vi "Genius_game_mvp1.vi"() -> ()   [LabVIEW 2020]
doc: "Use this template to build a simple state machine design pattern. Each state executes code and determines which state to transition to."
uses:
  controls/Data.ctl
  Control 1.ctl
  <vilib>/numeric/Random Number (Range) I64.vi
  <vilib>/numeric/sub_Random U32.vi
panel:
  in  "Cancel Button":bool
  out "?":i32
  in  "Play":bool
  in  "?":T1
  out "?":u32(colorbox)
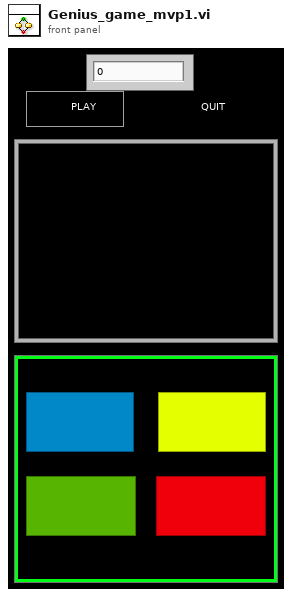
[diagram p1: front panel]
types:
  T1 = cluster{"BLUE":bool, "YELLOW":bool, "GREEN":bool, "RED":bool}
  T2 = typedef "Control 1.ctl" = enum32{"Play", "Initialise", "Create Colours", "Show colours sequence", "Wait for event", "pause", "Press colours sequence", "Compare colours", "Success ", "Failure", "Exit"}
  T3 = typedef "Data.ctl" = cluster{"Colours":i64[], "history ":i64[], "Wait time(ms)":u64, "String":string, "picked color":i64, "User's turn":i64, "Score":i64}
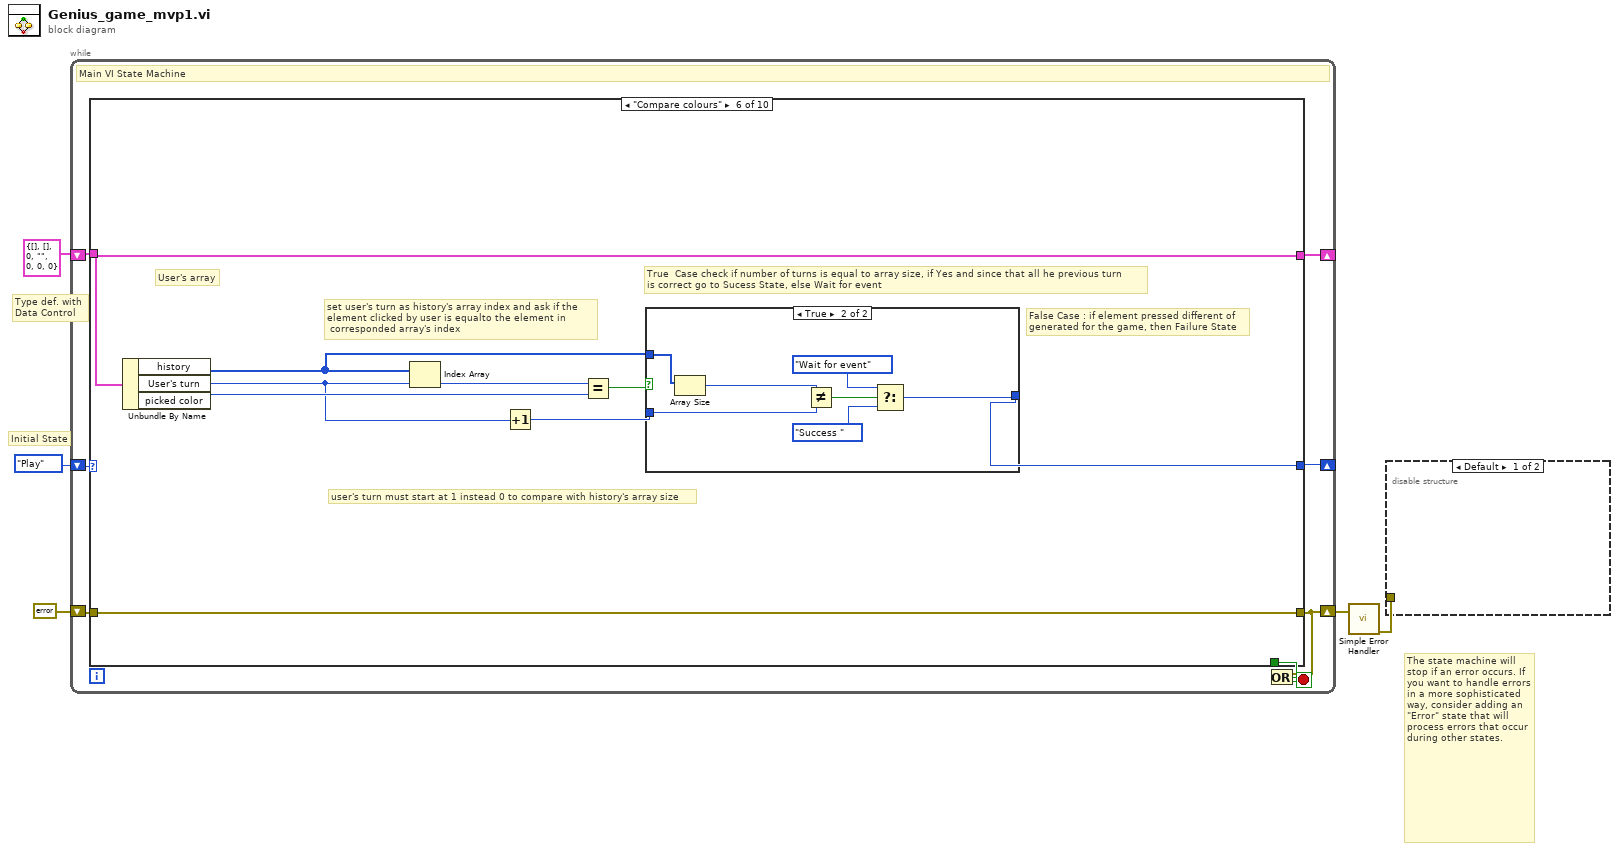
[diagram p0: block diagram]
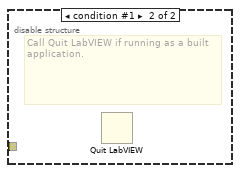
[diagram p2: hidden frame]
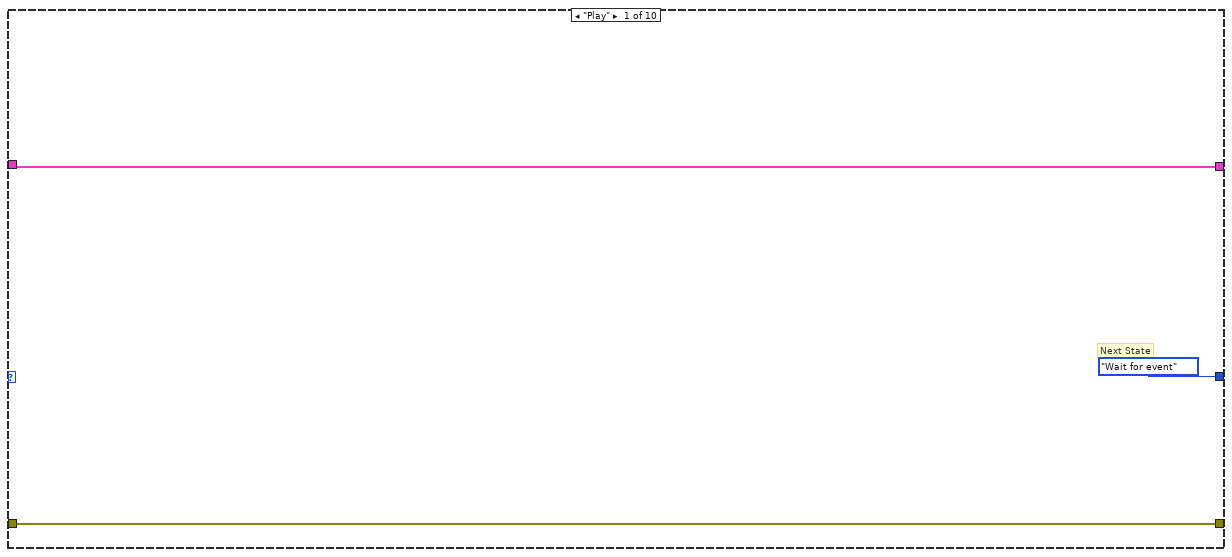
[diagram p3: hidden frame]
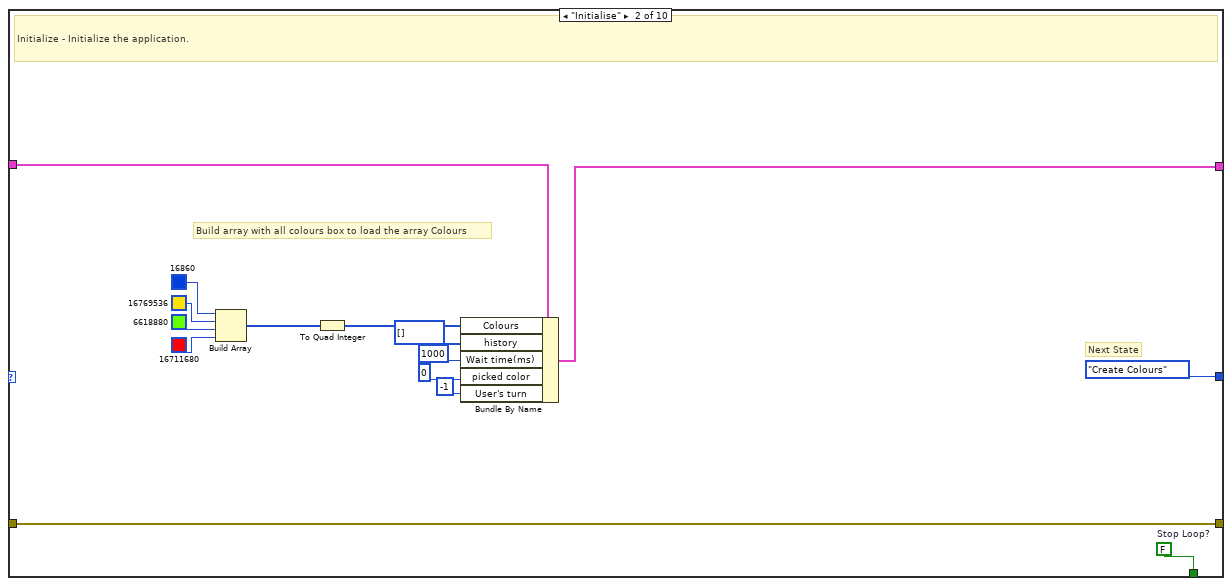
[diagram p4: hidden frame]
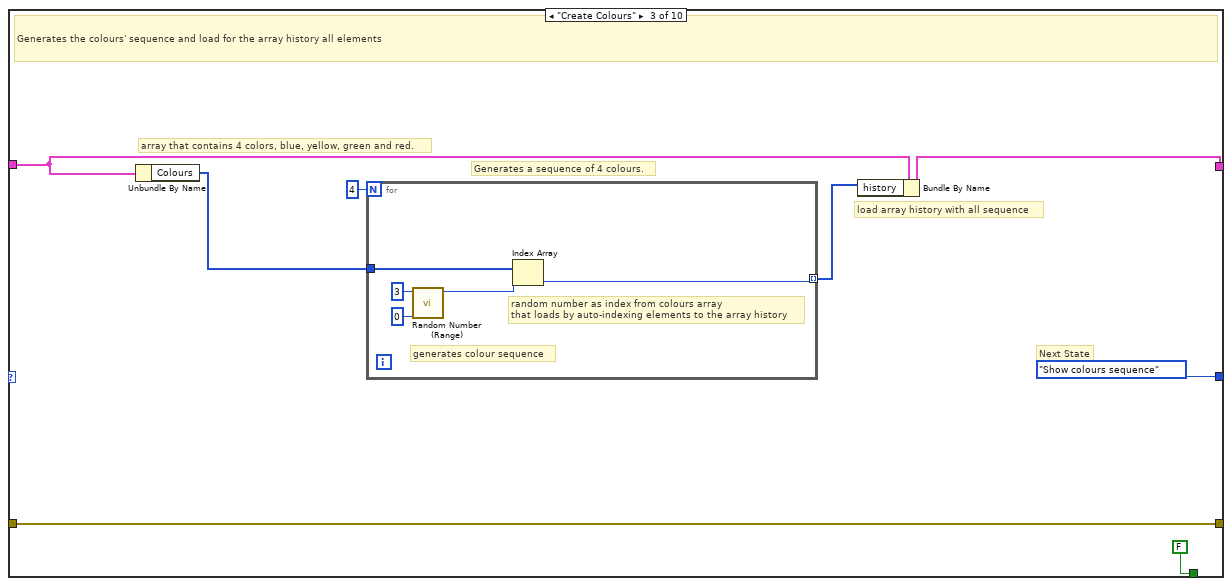
[diagram p5: hidden frame]
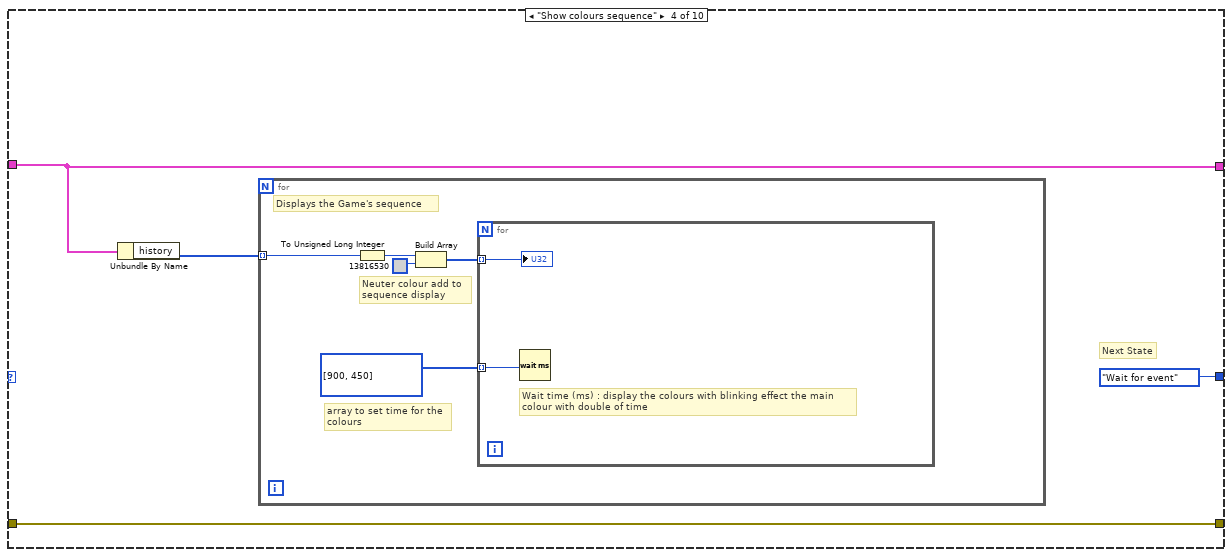
[diagram p6: hidden frame]
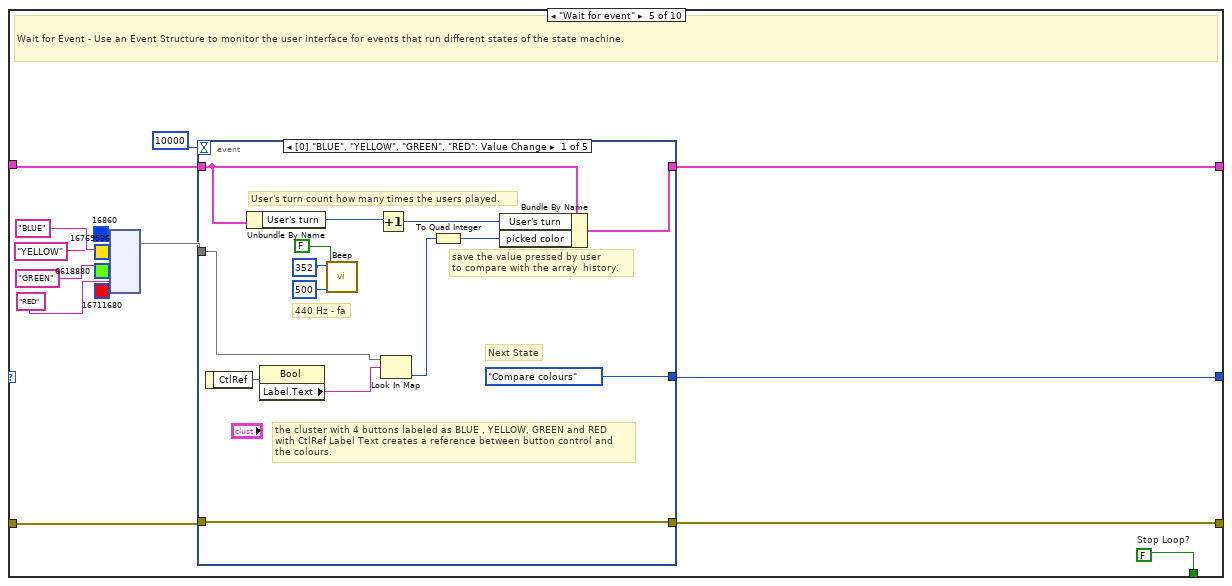
[diagram p7: hidden frame]
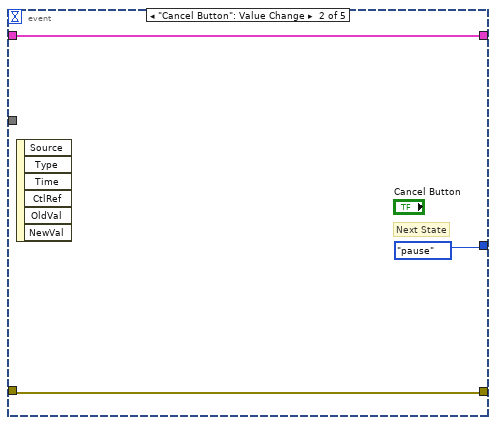
[diagram p8: hidden frame]
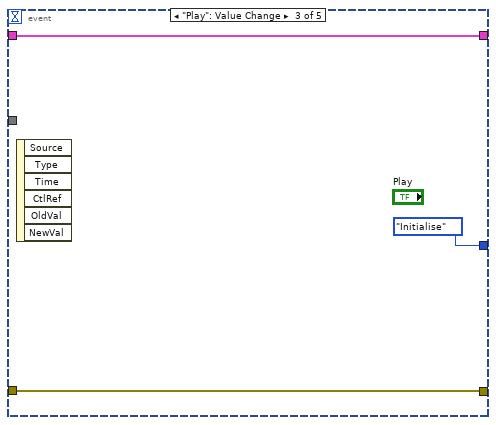
[diagram p9: hidden frame]
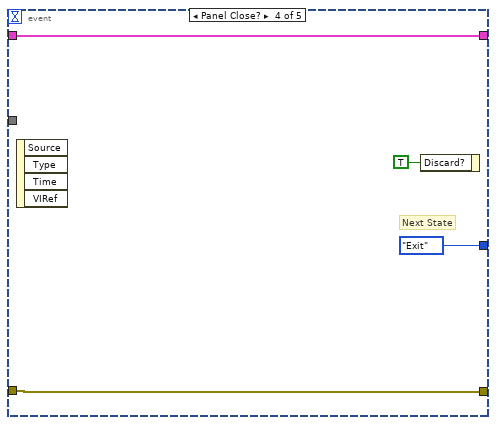
[diagram p10: hidden frame]
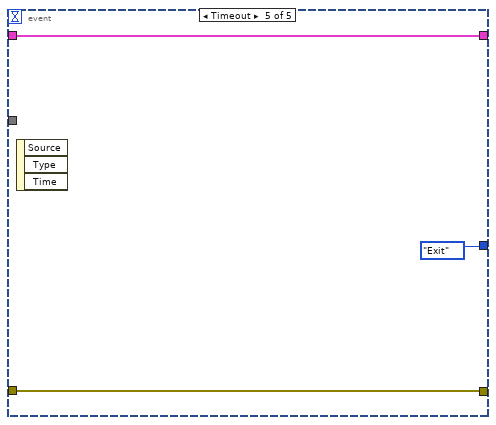
[diagram p11: hidden frame]
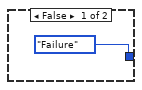
[diagram p12: hidden frame]
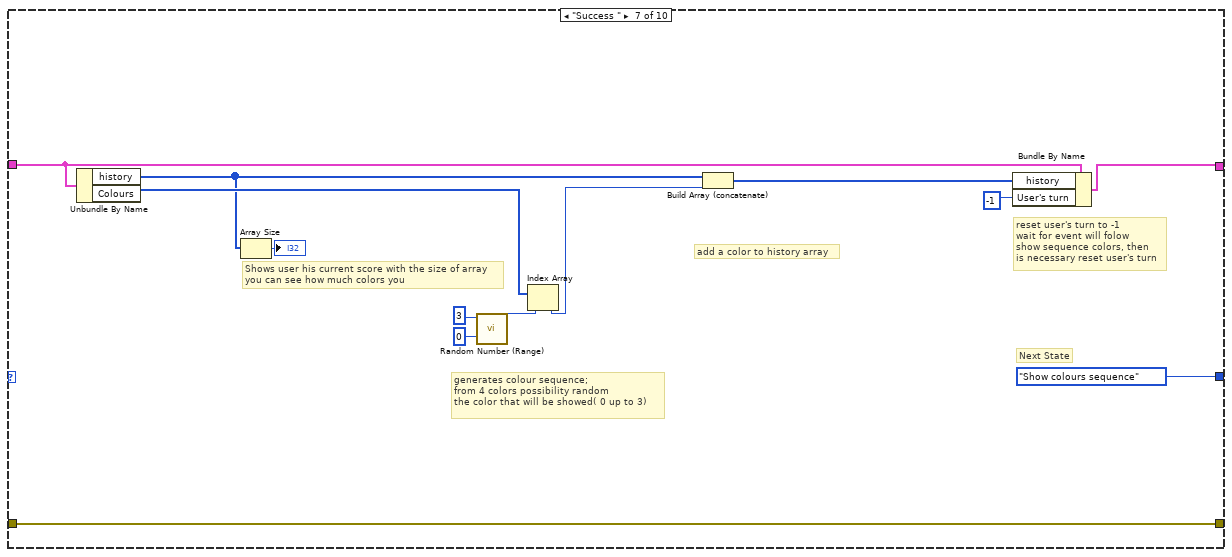
[diagram p13: hidden frame]
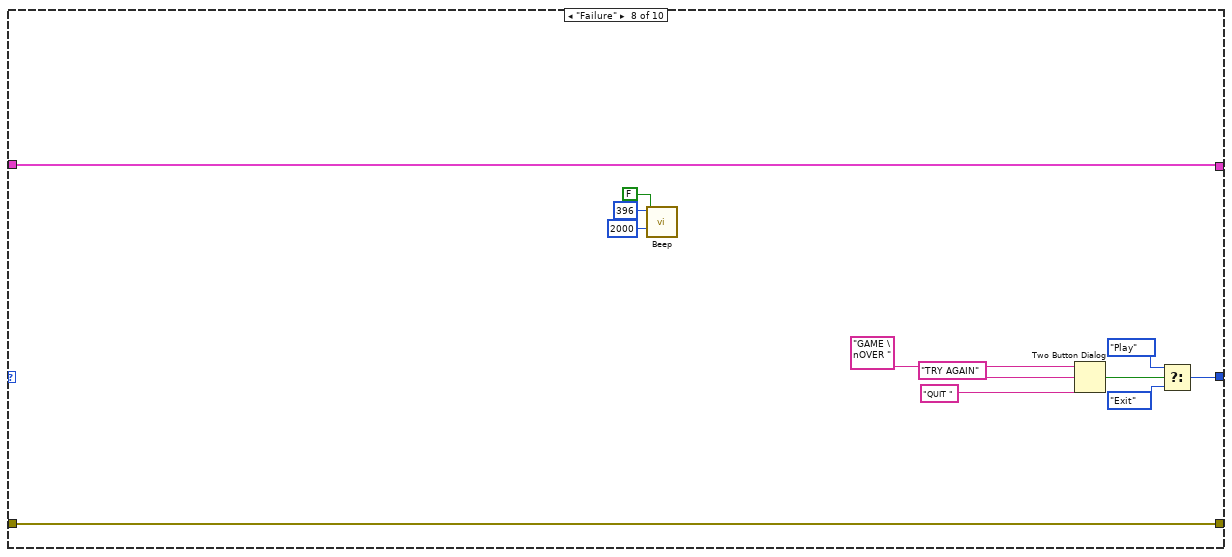
[diagram p14: hidden frame]
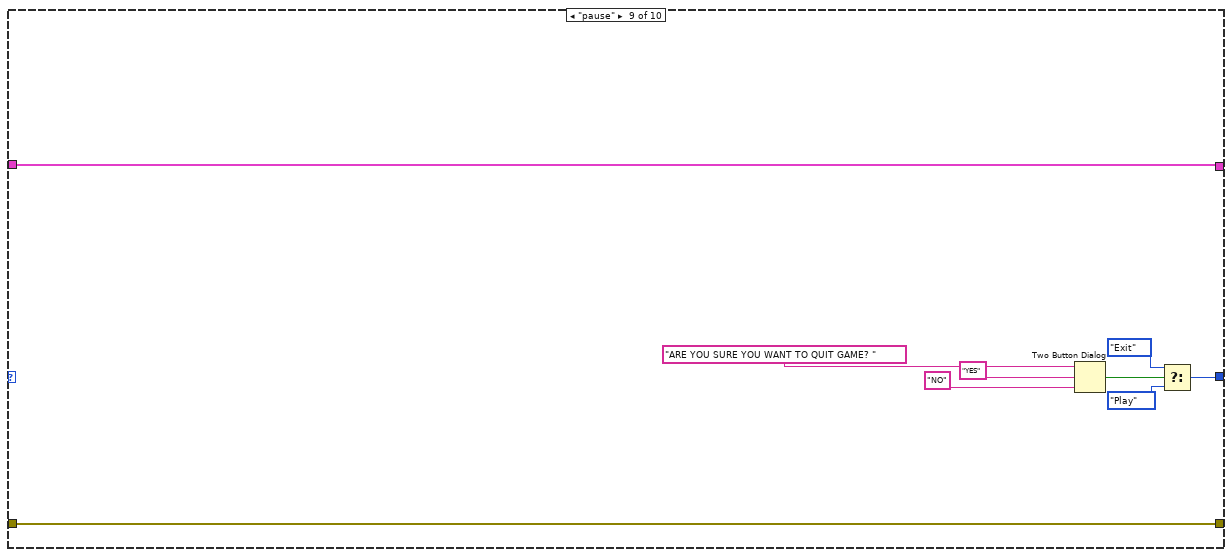
[diagram p15: hidden frame]
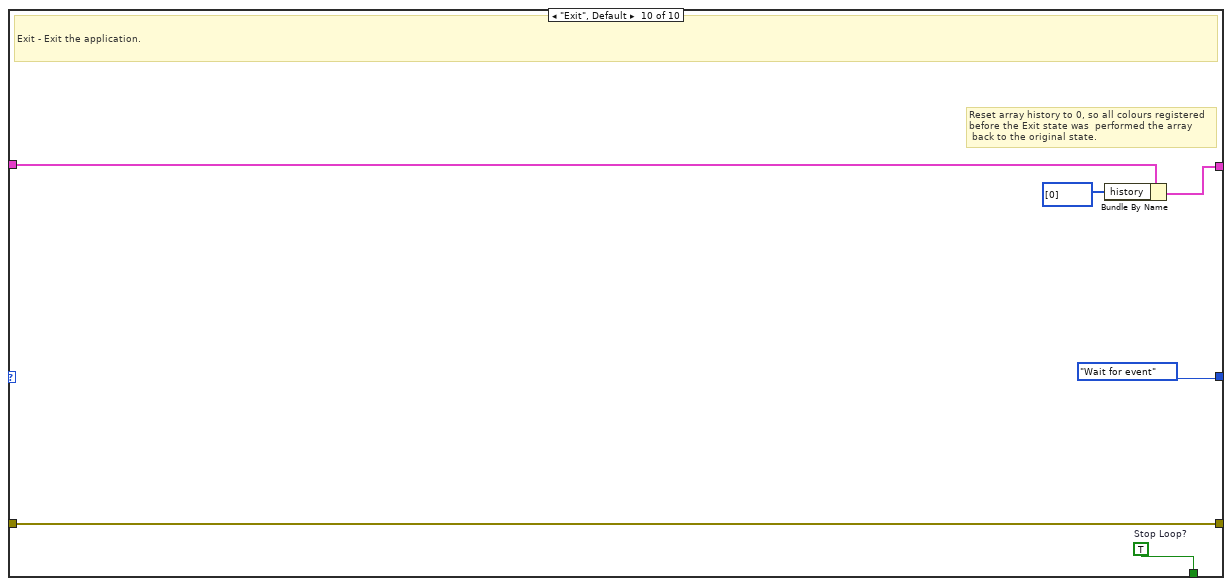
[diagram p16: hidden frame]
diagram:
  # "Type def. with\nData Control"
  # "Initial State"
  # "The state machine will stop if an error occurs. If you want to handle errors in a more sophisticated way, consider adding an \"Error\" state that will process errors that occur during other states."
  n1 = while {
    shift-right: [w12] -> _
    shift-left: T3 {"Colours"=[], "history "=[], "Wait time(ms)"=0, "String"="", "picked color"=0, "User's turn"=0, "Score"=0} ("Data") -> [w13]
    shift-right: [w9] -> w3
    shift-left: errorcluster {"status"=FALSE, "code"=0, "source"=""} ("error constant") -> [w11]
    shift-right: [w7] -> _
    shift-left: Control_1."Play" -> [w8]
    stop <- w10 stop-if-true
    # "Main VI State Machine"
    n2 = case shown="\"Compare colours\"" w8 {
      tunnel: [Control_1."Wait for event" Control_1."Create Colours" Control_1."Show colours sequence" Control_1."Wait for event" w59 w101 Control_1."Show colours sequence" w132 w143 Control_1."Wait for event"] -> w7
      tunnel: [_ w31 FALSE ("Stop Loop?") _ w71 _ _ _ _ w155] -> w6
      tunnel: w13 -> [w16 w29 w36 w47 w70 w106 w122 w140 w149 w151]
      tunnel: [w16 w28 w35 w47 w58 w106 w116 w140 w149 w153] -> w12
      tunnel: w11 -> [w15 w30 w38 w48 w56 w107 w128 w139 w148 w154]
      tunnel: [w15 w30 w38 w48 w69 w107 w128 w139 w148 w154] -> w9
      frame "Play" {
        # "Next State"
      }
      frame "Initialise" {
        w31 = FALSE  # Stop Loop?
        # "Next State"
        # "Build array with all colours box to load the array Colours"
        # "Initialize - Initialize the application."
        n3 = Build Array(u32 16860, u32 16769536, u32 6618880, u32 16711680) -> (w24:u32[])
        n4 = To Quad Integer(1:w24) -> (0:w23:i64[])
        n5 = Bundle By Name(cluster=w29, "Colours"=w23, "history"=i64[] [], "Wait time(ms)"=u64 1000, "picked color"=u64 0, "User's turn"=i64 -1) -> (w28:T3)
      }
      frame "Create Colours" {
        # "array that contains 4 colors, blue, yellow, green and red."
        # "Generates a sequence of 4 colours."
        # "Next State"
        # "load array history with all sequence"
        # "Generates the colours' sequence and load for the array history all elements"
        n6 = Unbundle By Name(w36) -> ("Colours"=w33:i64[])
        n7 = for {
          N: 4 -> [_]
          tunnel: w33 -> [w43]
          tunnel: [w44] -> w34 mode=indexing
          # "random number as index from colours array \nthat loads by auto-indexing elements to the array history"
          # "generates colour sequence"
          n8 = call-poly <vilib>:"Random Number (Range).vi"("lower bound (-100)"=i64 0, "upper bound (100)"=i64 3) -> ("number"=w40:i64)  [unwired: 9 in]
          n9 = Index Array(array=w43, index=w40) -> (element=w44:i64)
        }
        n10 = Bundle By Name(cluster=w36, "history"=w34) -> (w35:T3)
      }
      frame "Show colours sequence" {
        # "Next State"
        n11 = Unbundle By Name(w47) -> ("history"=w46:i64[])
        n12 = for {
          tunnel: w46 -> [w51] mode=indexing
          # "Neuter colour add to\nsequence display"
          # "array to set time for the \ncolours"
          # "Displays the Game's sequence"
          n13 = To Unsigned Long Integer(number=w51) -> (unsigned 32bit integer=w50:u32)
          n14 = Build Array(w50, u32 13816530) -> (w53:u32[])
          n15 = for {
            tunnel: w53 -> [w55] mode=indexing
            tunnel: u32[] [900, 450] ("millisecond timer value") -> [w54] mode=indexing
            # "Wait time (ms) : display the colours with blinking effect the main \ncolour with double of time"
            n16 = Wait (ms)(milliseconds to wait=w54) -> ()  [unwired: 1 out]
            "?" <- w55
          }
        }
      }
      frame "Wait for event" {
        w71 = FALSE  # Stop Loop?
        # "Wait for Event - Use an Event Structure to monitor the user interface for events that run different states of the state machine."
        n17 = node("BLUE" ("key"), u32 16860, "YELLOW" ("key"), u32 16769536, "GREEN" ("key"), u32 6618880, "RED" ("key"), u32 16711680) -> (w60:map{string, u32})
        n18 = event shown="[0] \"BLUE\", \"YELLOW\", \"GREEN\", \"RED\": Value Change" {
          selector: _ -> [_ _ _ _ _]
          dyn-events: _ -> [_ _ _ _ _]
          timeout: 10000 -> [_ _ _ _ _]
          tunnel: w70 -> [w81 w87 w90 w94 w97]
          tunnel: [w75 w88 w91 w95 w98] -> w69
          tunnel: w60 -> [w83 _ _ _ _]
          tunnel: [Control_1."Compare colours" ("f") Control_1."pause" Control_1."Initialise" Control_1."Exit" Control_1."Exit"] -> w59
          tunnel: [w80 w87 w90 w94 w97] -> w58
          tunnel: w56 -> [w75 w88 w91 w95 w98]
          event Value Change {
            # "440 Hz - fa"
            # "save the value pressed by user\nto compare with the array  history."
            # "User's turn count how many times the users played."
            # "the cluster with 4 buttons labeled as BLUE , YELLOW, GREEN and RED\nwith CtlRef Label Text creates a reference between button control and\nthe colours."
            # "Next State"
            n19 = event-data() -> ("CtlRef"=w85:refnum<vi>)  [unwired: 1 in]
            n20 = Unbundle By Name(w81) -> ("User's turn"=w79:i64)
            n21 = property class="Bool"(reference=w85) -> ("Label.Text"=w84:string)  [unwired: 1 in, 2 out]
            n22 = call <vilib>:"Beep.vi"("use system alert? (T)"=FALSE, "duration (msec)"=u32 500, "frequency (Hz)"=u32 352) -> ()  [unwired: 9 in]
            n23 = Increment(x=w79) -> (x+1=w78:i64)
            n24 = Look In Map(map=w83, key=w84) -> (value=w77:u32)  [unwired: 1 in, 1 out]
            n25 = To Quad Integer(1:w77) -> (0:w76:i64)
            n26 = Bundle By Name(cluster=w81, "User's turn"=w78, "picked color"=w76) -> (w80:T3)
          }
          event "Cancel Button": Value Change {
            # "Next State"
            n27 = event-data() -> ()  [unwired: 1 in, 6 out]
          }
          event "Play": Value Change {
            n28 = event-data() -> ()  [unwired: 1 in, 6 out]
          }
          event Panel Close? {
            # "Next State"
            n29 = event-data() -> ()  [unwired: 1 in, 4 out]
            n30 = event-data("Discard?"=TRUE) -> ()  [unwired: 1 in, 1 out]
          }
          event Timeout {
            n31 = event-data() -> ()  [unwired: 1 in, 3 out]
          }
        }
      }
      frame "Compare colours" {
        # "False Case : if element pressed different of\ngenerated for the game, then Failure State"
        # "True  Case check if number of turns is equal to array size, if Yes and since that all he previous turn\nis correct go to Sucess State, else Wait for event"
        # "set user's turn as history's array index and ask if the \nelement clicked by user is equalto the element in\n corresponded array's index"
        # "user's turn must start at 1 instead 0 to compare with history's array size"
        # "User's array"
        n32 = Unbundle By Name(w106) -> ("history"=w102:i64[], "User's turn"=w99:i64, "picked color"=w105:i64)
        n33 = Index Array(array=w102, index=w99) -> (element=w104:i64)
        n34 = Increment(x=w99) -> (x+1=w100:i64)
        n35 = Equal?(x=w104, y=w105) -> (x = y?=w103:bool)
        n36 = case shown="True" w103 {
          tunnel: w102 -> [_ w115]
          tunnel: [Control_1."Failure" w111] -> w101
          tunnel: w100 -> [_ w109]
          frame False {
          }
          frame True {
            n37 = Array Size(array=w115) -> (size(s)=w110:i32)
            n38 = Not Equal?(x=w110, y=w109) -> (x != y?=w114:bool)
            n39 = Select(t=Control_1."Wait for event", s=w114, f=Control_1."Success ") -> (s? t:f=w111:T2)
          }
        }
      }
      frame "Success " {
        # "Shows user his current score with the size of array\nyou can see how much colors you"
        # "Next State"
        # "reset user's turn to -1\nwait for event will folow \nshow sequence colors, then \nis necessary reset user's turn"
        # "add a color to history array"
        # "generates colour sequence;\nfrom 4 colors possibility random \nthe color that will be showed( 0 up to 3)"
        n40 = Unbundle By Name(w122) -> ("history"=w117:i64[], "Colours"=w126:i64[])
        n41 = Array Size(array=w117) -> (size(s)=→"?":i32)
        n42 = call-poly <vilib>:"Random Number (Range).vi"("lower bound (-100)"=i64 0, "upper bound (100)"=i64 3) -> ("number"=w123:i64)  [unwired: 9 in]
        n43 = Index Array(array=w126, index=w123) -> (element=w121:i64)
        n44 = Build Array (concatenate)(w117, w121) -> (w119:i64[])
        n45 = Bundle By Name(cluster=w122, "history"=w119, "User's turn"=i64 -1) -> (w116:T3)
      }
      frame "Failure" {
        n46 = call <vilib>:"Beep.vi"("use system alert? (T)"=FALSE, "duration (msec)"=u32 2000, "frequency (Hz)"=u32 396) -> ()  [unwired: 9 in]
        n47 = Two Button Dialog(message="GAME \nOVER ", 1:"QUIT " ("F button name (\"Cancel\")"), 2:"TRY AGAIN" ("T button name (\"OK\")")) -> (T button?=w135:bool)
        n48 = Select(t=Control_1."Play", s=w135, f=Control_1."Exit") -> (s? t:f=w132:T2)
      }
      frame "pause" {
        n49 = Two Button Dialog(message="ARE YOU SURE YOU WANT TO QUIT GAME? ", 1:"NO" ("F button name (\"Cancel\")"), 2:"YES" ("T button name (\"OK\")")) -> (T button?=w146:bool)
        n50 = Select(t=Control_1."Exit", s=w146, f=Control_1."Play") -> (s? t:f=w143:T2)
      }
      frame "Exit", Default {
        w155 = TRUE  # Stop Loop?
        # "Reset array history to 0, so all colours registered\nbefore the Exit state was  performed the array\n back to the original state."
        # "Exit - Exit the application."
        n51 = Bundle By Name(cluster=w151, "history"=i64[] [0]) -> (w153:T3)
      }
    }
    n52 = Or(x=w9, y=w6) -> (x .or. y?=w10:bool)
  }
  n53 = call <vilib>:"Simple Error Handler.vi"("error in (no error)"=w3) -> ("error out"=w2:errorcluster)  [unwired: 4 in, 4 out]
  n54 = disable-structure shown="Default" {
    disable-tunnel: w2 -> [_ _]
    frame condition #0 (active) {
    }
    frame condition #1 {
      # "Call Quit LabVIEW if running as a built application."
      n55 = Quit LabVIEW() -> ()  [unwired: 1 in]
    }
  }
